vi "ROI Barycenter.vi"(8 "Error In":errorcluster, 11 "ROI Descriptor in":T1 {"Contours"."Type" items=["No Selection", "Point", "Line", "Rectangle", "Oval", "Polygon", "Freehand Region", "Annulus", "Unused2", "Unused3", "Broken Line", "Freehand Line", "Rotated Rectangle"]}) -> (0 "Error Out":errorcluster, 3 "ROI Center":cluster{"X":dbl, "Y":dbl})   [LabVIEW 2021, in "Image.lvlib"]
uses:
  Image.lvlib
  <vilib>/Utility/error.llb/Error Cluster From Error Code.vi
  <vilib>/ErrorRing/Error Ring.xnode
  Math/Math.lvlib
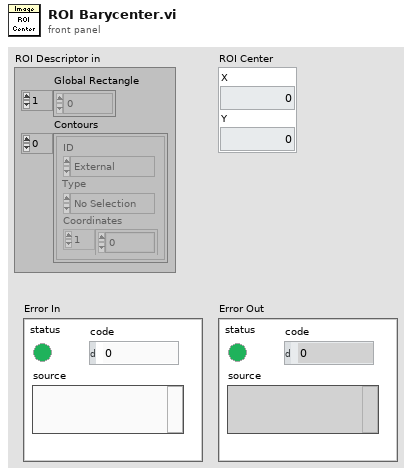
[diagram p1: front panel]
types:
  T1 = typedef "ROI Descriptor" = cluster{"Global Rectangle":i32[], "Contours":cluster{"ID":enum32{"External", "Internal"}, "Type":u32, "Coordinates":i32[]}[]}
  T2 = cluster{"ID":enum32{"External", "Internal"}, "Type":u32, "Coordinates":i32[]}[]
  T3 = cluster{"ID":enum32{"External", "Internal"}, "Type":u32, "Coordinates":i32[]}
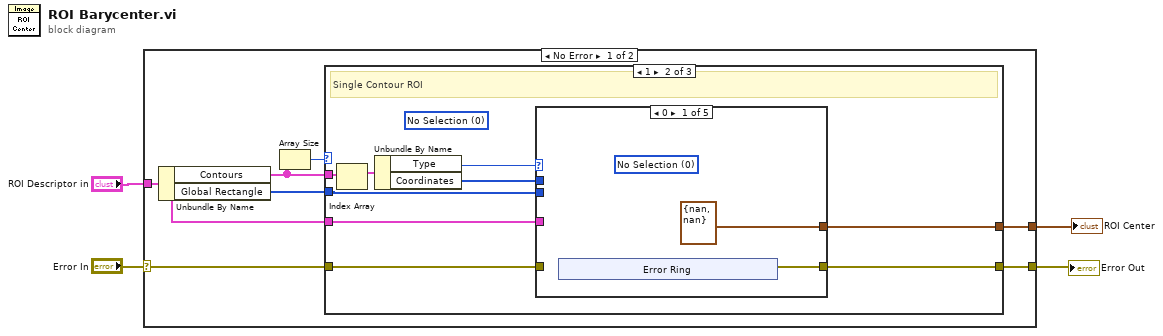
[diagram p0: block diagram]
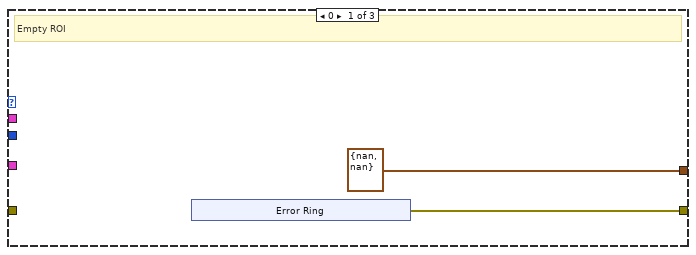
[diagram p2: hidden frame]
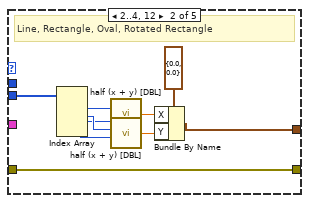
[diagram p3: hidden frame]
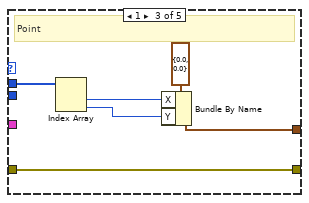
[diagram p4: hidden frame]
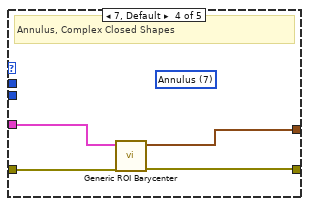
[diagram p5: hidden frame]
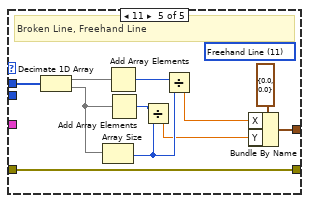
[diagram p6: hidden frame]
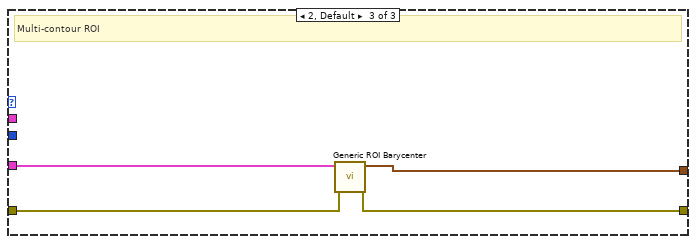
[diagram p7: hidden frame]
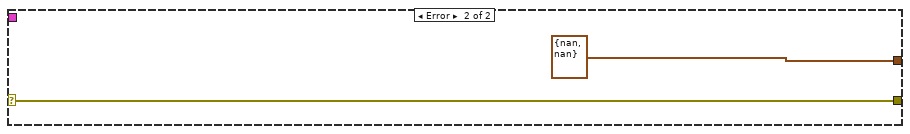
[diagram p8: hidden frame]
diagram:
  n1 = case shown="No Error" "Error In" {
    selector: "Error In" -> [w6 w69]
    tunnel: [w10 cluster{"X":dbl, "Y":dbl} {"X"=nan, "Y"=nan} ("ROI Center")] -> w4
    tunnel: "ROI Descriptor in" -> [w5 _]
    tunnel: [w7 w69] -> w1
    frame No Error {
      n2 = Unbundle By Name(w5) -> ("Contours"=w9:T2, "Global Rectangle"=w11:i32[])
      n3 = Array Size(array=w9) -> (size(s)=w8:i32)
      n4 = case shown="1" w8 {
        tunnel: w11 -> [_ w26 _]
        tunnel: [cluster{"X":dbl, "Y":dbl} {"X"=nan, "Y"=nan} ("ROI Center") w25 w64] -> w10
        tunnel: w9 -> [_ w23 _]
        tunnel: [w12 w21 w65] -> w7
        tunnel: w6 -> [_ w20 w66]
        tunnel: w5 -> [_ w18 w67]
        frame 0 {
          # "Empty ROI"
          n5 = xnode "Error Ring"() -> ("error out"=w12:errorcluster)
        }
        frame 1 {
          (unwired) u32 0 items=["No Selection", "Point", "Line", "Rectangle", "Oval", "Polygon", "Freehand Region", "Annulus", "Unused2", "Unused3", "Broken Line", "Freehand Line", "Rotated Rectangle"] ("Type")
          # "Single Contour ROI"
          n6 = Index Array(array=w23) -> (element=w24:T3)  [unwired: 1 in]
          n7 = Unbundle By Name(w24) -> ("Type"=w22:u32, "Coordinates"=w19:i32[])
          n8 = case shown="0" w22 {
            tunnel: w26 -> [_ w36 _ _ _]
            tunnel: [cluster{"X":dbl, "Y":dbl} {"X"=nan, "Y"=nan} ("ROI Center") w35 w48 w49 w61] -> w25
            tunnel: [w27 w33 w46 w50 w53] -> w21
            tunnel: w20 -> [_ w33 w46 w51 w53]
            tunnel: w19 -> [_ _ w43 _ w63]
            tunnel: w18 -> [_ _ _ w52 _]
            frame 0 {
              (unwired) u32 0 items=["No Selection", "Point", "Line", "Rectangle", "Oval", "Polygon", "Freehand Region", "Annulus", "Unused2", "Unused3", "Broken Line", "Freehand Line", "Rotated Rectangle"] ("Type")
              n9 = xnode "Error Ring"() -> ("error out"=w27:errorcluster)
            }
            frame 2..4, 12 {
              # "Line, Rectangle, Oval,\tRotated Rectangle"
              n10 = Index Array(array=w36) -> (element #1=w37:i32, element #2=w40:i32, element #3=w38:i32, element #4=w41:i32)  [unwired: 4 in]
              n11 = call "half (x + y) [DBL].vi"("y"=w38, "x"=w37) -> ("(x+y)/2"=w39:dbl)  [unwired: 4 in]
              n12 = call "half (x + y) [DBL].vi"("y"=w41, "x"=w40) -> ("(x+y)/2"=w42:dbl)  [unwired: 4 in]
              n13 = Bundle By Name(cluster=cluster{"X":dbl, "Y":dbl} {"X"=0.0, "Y"=0.0} ("ROI Center"), "X"=w39, "Y"=w42) -> (w35:cluster{"X":dbl, "Y":dbl})
            }
            frame 1 {
              # "Point"
              n14 = Index Array(array=w43) -> (element #1=w45:i32, element #2=w44:i32)  [unwired: 2 in]
              n15 = Bundle By Name(cluster=cluster{"X":dbl, "Y":dbl} {"X"=0.0, "Y"=0.0} ("ROI Center"), "X"=w45, "Y"=w44) -> (w48:cluster{"X":dbl, "Y":dbl})
            }
            frame 7, Default {
              (unwired) u32 7 items=["No Selection", "Point", "Line", "Rectangle", "Oval", "Polygon", "Freehand Region", "Annulus", "Unused2", "Unused3", "Broken Line", "Freehand Line", "Rotated Rectangle"] ("Type")
              # "Annulus, Complex Closed Shapes"
              n16 = call "Generic ROI Barycenter.vi"("error in (no error)"=w51, "ROI Descriptor"=w52) -> ("error out"=w50:errorcluster, "ROI Center"=w49:cluster{"X":dbl, "Y":dbl})  [unwired: 8 in]
            }
            frame 11 {
              (unwired) u32 11 items=["No Selection", "Point", "Line", "Rectangle", "Oval", "Polygon", "Freehand Region", "Annulus", "Unused2", "Unused3", "Broken Line", "Freehand Line", "Rotated Rectangle"] ("Type")
              # "Broken Line, Freehand Line"
              n17 = Decimate 1D Array(w63) -> (w60:i32[], w59:i32[])
              n18 = Array Size(array=w59) -> (size(s)=w55:i32)
              n19 = Add Array Elements(numeric array=w60) -> (sum=w58:i32)
              n20 = Add Array Elements(numeric array=w59) -> (sum=w56:i32)
              n21 = Divide(x=w56, y=w55) -> (x/y=w54:dbl)
              n22 = Divide(x=w58, y=w55) -> (x/y=w57:dbl)
              n23 = Bundle By Name(cluster=cluster{"X":dbl, "Y":dbl} {"X"=0.0, "Y"=0.0} ("ROI Center"), "X"=w57, "Y"=w54) -> (w61:cluster{"X":dbl, "Y":dbl})
            }
          }
        }
        frame 2, Default {
          # "Multi-contour ROI"
          n24 = call "Generic ROI Barycenter.vi"("error in (no error)"=w66, "ROI Descriptor"=w67) -> ("error out"=w65:errorcluster, "ROI Center"=w64:cluster{"X":dbl, "Y":dbl})  [unwired: 8 in]
        }
      }
    }
    frame Error {
    }
  }
  "ROI Center" <- w4
  "Error Out" <- w1
